vi "configuration UI.vi"() -> ()   [LabVIEW 2013, in "TEC editor node.lvclass"]
uses:
  TEC editor node.lvclass
  <vilib>/NI/Configuration Framework/Node/NodeRef.ctl
  <vilib>/NI/Configuration Framework/Node/NISE_CEF_Node.lvclass
  <vilib>/NI/AMC/Message Queue.ctl
  <vilib>/NI/AMC/Message.ctl
  <vilib>/NI/Tools/Keyed Array/KeyedArray.ctl
  <vilib>/NI/Configuration Framework/Node/UserEventRef.ctl
  <vilib>/NI/Configuration Framework/Controls/EventCluster.ctl
  <vilib>/NI/DCAF UI Toolkit/Controls/Move One Right.ctl
  <vilib>/NI/DCAF UI Toolkit/Controls/Move One Left.ctl
  configuration/TEC configuration.lvclass
  <vilib>/Utility/miscctls.llb/LVRowAndColumnTypeDef.ctl
  <vilib>/Utility/miscctls.llb/LVPositionTypeDef.ctl
  configuration/TEC configuration.lvclass/TEC configuration.ctl
  TEC editor node.lvclass/TEC editor node.ctl
  <vilib>/NI/Tag Bus/tag/Data Type.ctl
  <vilib>/NI/Tag Bus Module Framework/channel/channel classification.ctl
  <vilib>/NI/Tag Bus Module Framework/channel/TBM channel.lvclass/TBM channel.ctl
  <vilib>/NI/Configuration Framework/serializable configuration/NISE_CEF_serializable configuration.lvclass/NISE_CEF_serializable configuration.ctl
  <vilib>/NI/Tag Bus/tag/tag descriptor.lvclass/tag descriptor.ctl
  configuration/Write receive on port.vi
  configuration/Write send to port.vi
  configuration/Write send from port.vi
  configuration/Write send to address.vi
  configuration/Write estimated array size.vi
  configuration/Read receive on port.vi
  configuration/Read send from port.vi
  configuration/Read send to address.vi
  configuration/Read send to port.vi
  configuration/Read estimated array size.vi
  <vilib>/NI/DCAF/Tag Editor Core/Configuration Editor/Classes/Module editor node/Read display name.vi
  <vilib>/Utility/LVClass/Get LV Class Name.vi
  <vilib>/NI/Configuration Framework/error generator/NISE_error generator.vi
  <vilib>/NI/Configuration Framework/serializable configuration/NISE_CEF_serializable configuration.lvclass
  <vilib>/NI/DCAF/Tag Editor Core/Configuration Editor/Classes/Module editor node/module editor node.lvclass
  <vilib>/NI/Configuration Framework/NISE_CEF_TreeControl.lvlib
  <vilib>/NI/Tag Bus/tag/tag descriptor.lvclass
  <vilib>/NI/Module Execution Interface/Engine Configuration/engine configuration.lvclass
  <vilib>/NI/Tag Bus Module Framework/channel/TBM channel.lvclass
  <vilib>/NI/DCAF/Tag Editor Core/Configuration Editor/Classes/Engine Parent/Engine Parent Editor Node.lvclass
  <vilib>/NI/DCAF UI Toolkit/Controls/DCAF UI Elements.lvlib
  <vilib>/NI/Tools/Keyed Array/Tools_KeyedArray.lvlib
  <vilib>/NI/AMC/AMC.lvlib
panel:
  in  "Tab Control":T1(tab)
  out "Guid":string
  in  "unpair":bool
  out "Paired with":string
  in  "pair":bool
  in  "Pairing Options":i32(listbox)
  in  "Filtering":string
  in  "remove to":T2
  in  "add to":T3
  in  "toExtList":i32(listbox)
  in  "fromExternallist":i32(listbox)
  in  "avail tags":i32(listbox)=-1
  in  "Estimated Received Array Size (bytes)":u16
  in  "receive on port":u16
  in  "send from port":u16
  in  "send to address":string
  in  "send to port":u16
  in  "user event":T4
  in  "main queue":T5
  in  "node ref":T6
  # "UDP Port Settings"
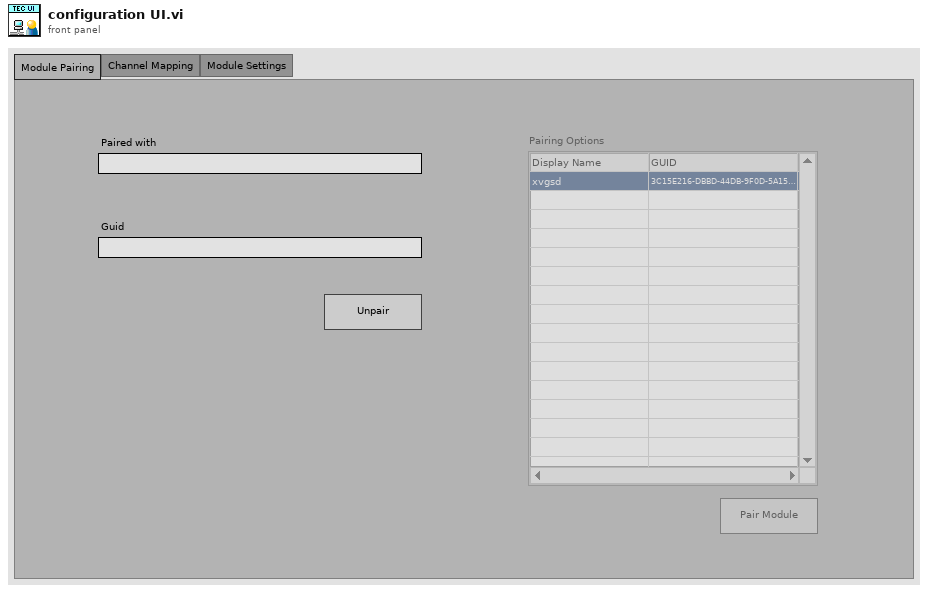
[diagram p1: front panel]
types:
  T1 = enum32{"Module Pairing", "Channel Mapping", "Module Settings"}
  T2 = typedef "DCAF UI Elements.lvlib/Move One Left.ctl" = bool
  T3 = typedef "DCAF UI Elements.lvlib/Move One Right.ctl" = bool
  T4 = typedef "NISE_CEF_Node.lvclass/UserEventRef.ctl" = refnum<user-event>
  T5 = typedef "AMC.lvlib/Message Queue.ctl" = refnum<queue>
  T6 = typedef "NISE_CEF_Node.lvclass/NodeRef.ctl" = refnum<data-value>
  T7 = typedef "LVPositionTypeDef.ctl" = cluster{"Left":i32, "Top":i32}
  T8 = typedef "LVRowAndColumnTypeDef.ctl" = cluster{"Row":i32, "Column":i32}
  T9 = typedef "NISE_CEF_TreeControl.lvlib/EventCluster.ctl" = cluster{"command":string, "data":string}
  T10 = typedef "TBM channel.lvclass/channel classification.ctl" = enum16{"input data", "output data", "processing parameter", "processing result"}
  T11 = typedef "tag bus.lvlib/tag descriptor.lvclass/Data Type.ctl" = enum16{"Double", "Single", "I64", "I32", "I16", "I8", "U64", "U32", "U16", "U8", "Boolean", "String", "Array of Double", "Array of Single", "Array of I64", "Array of I32", "Array of I16", "Array of I8", "Array of U64", "Array of U32", "Array of U16", "Array of U8", "Array of Boolean", "Array of String"}
  T12 = typedef "TEC editor node.lvclass/pair information.ctl" = cluster{"paired guid":string}
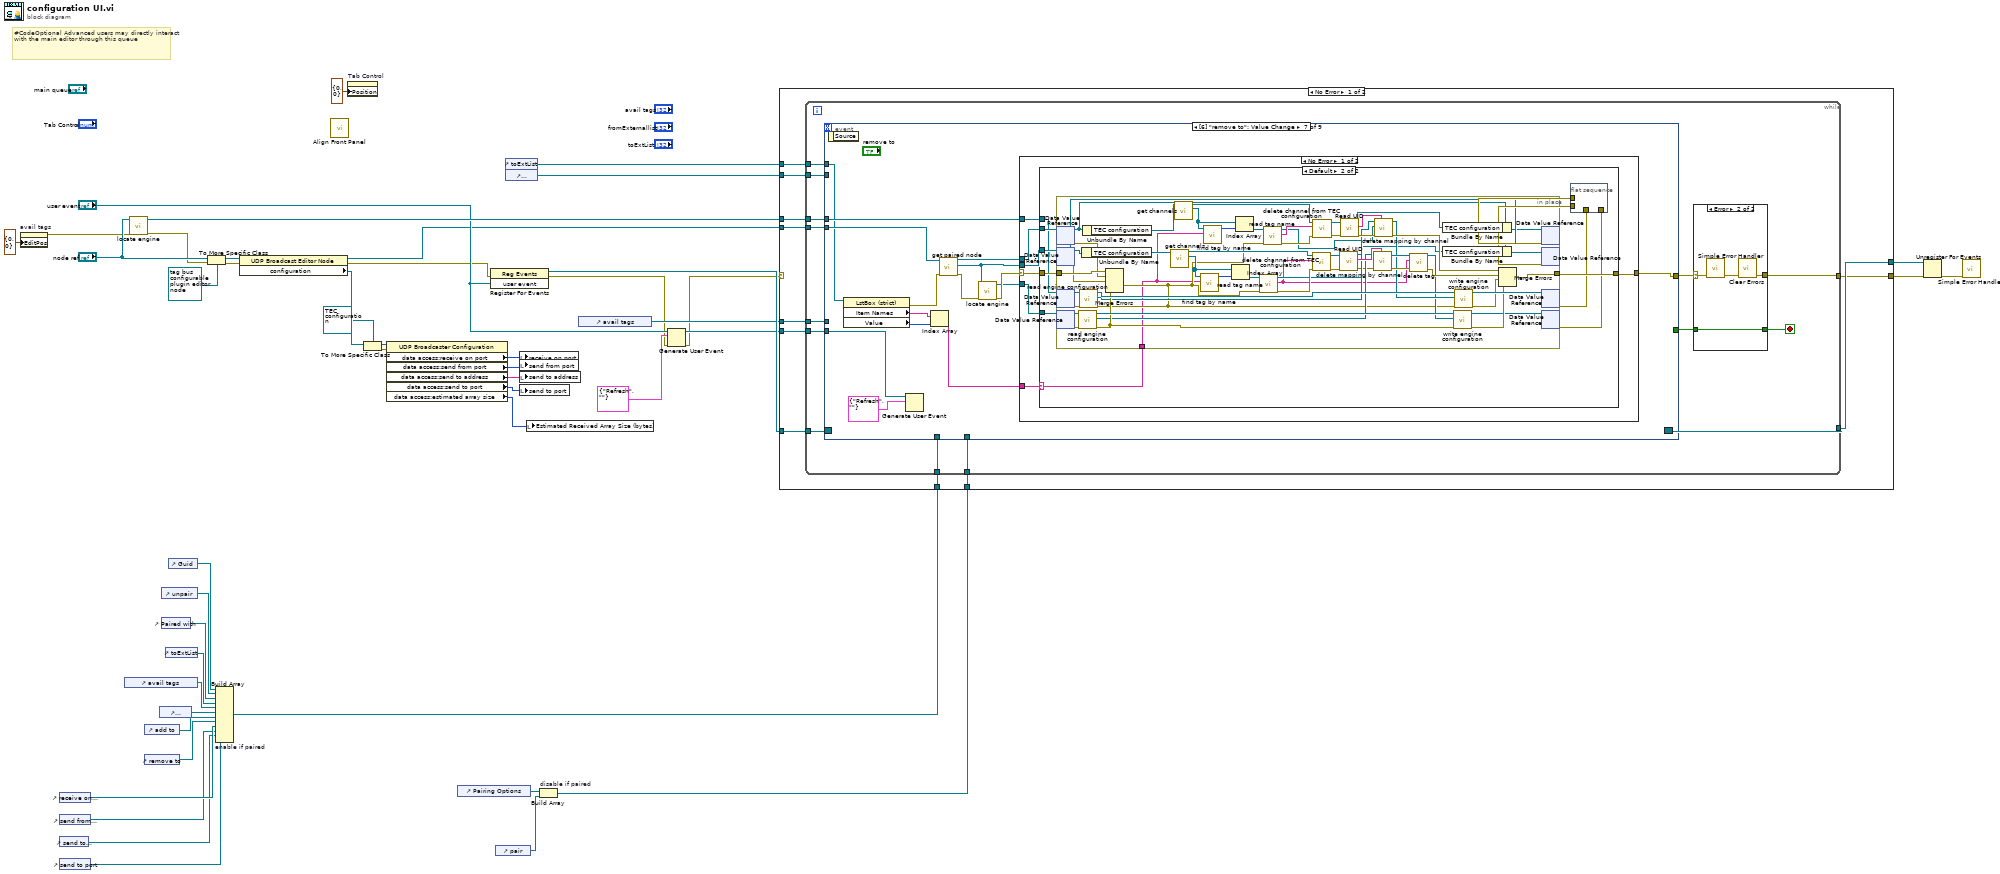
[diagram p0: block diagram]
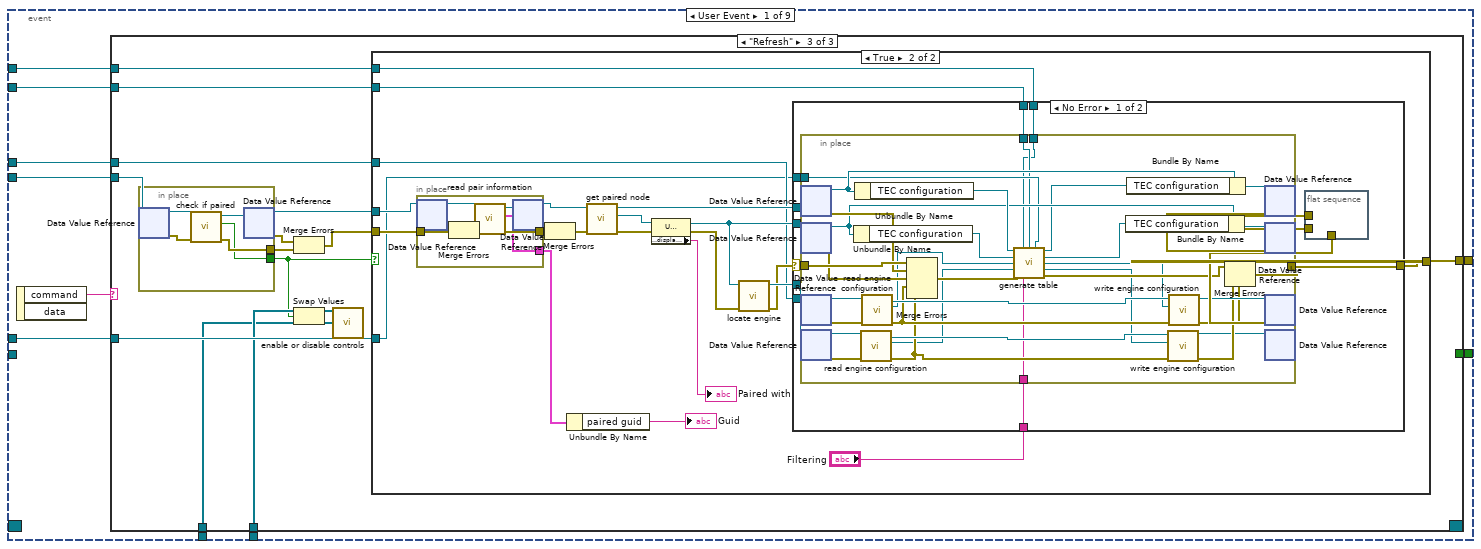
[diagram p3: hidden frame]
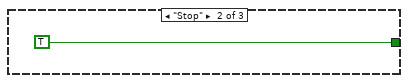
[diagram p5: hidden frame]
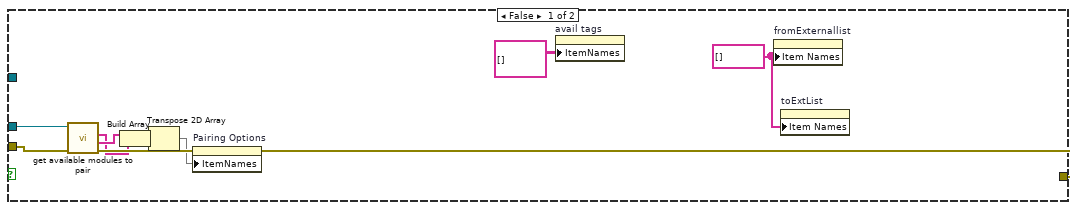
[diagram p6: hidden frame]
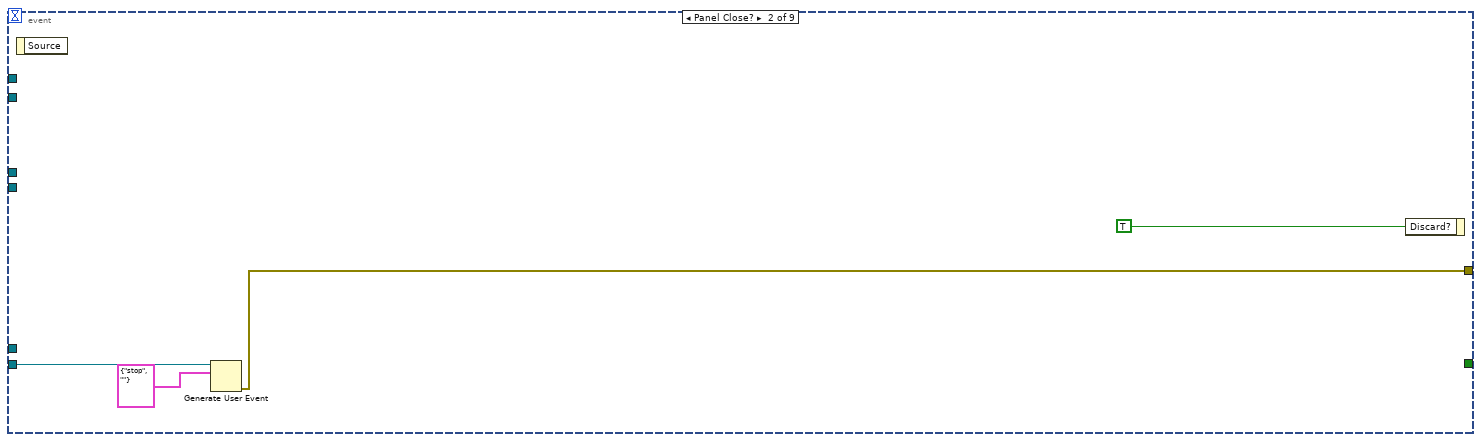
[diagram p8: hidden frame]
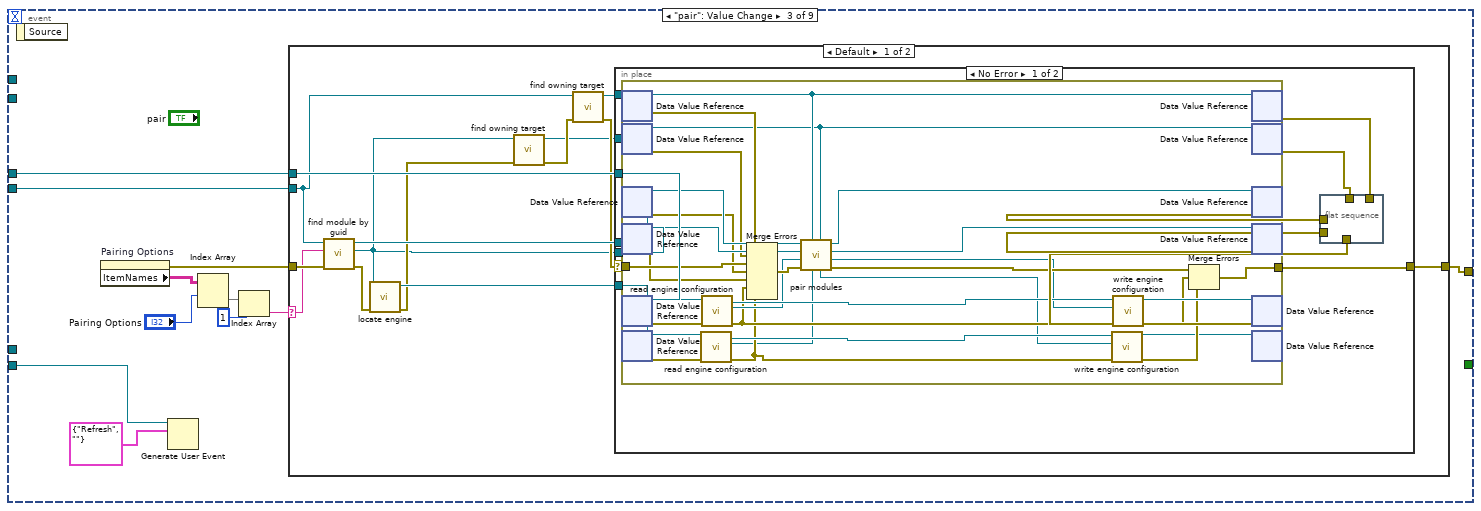
[diagram p9: hidden frame]
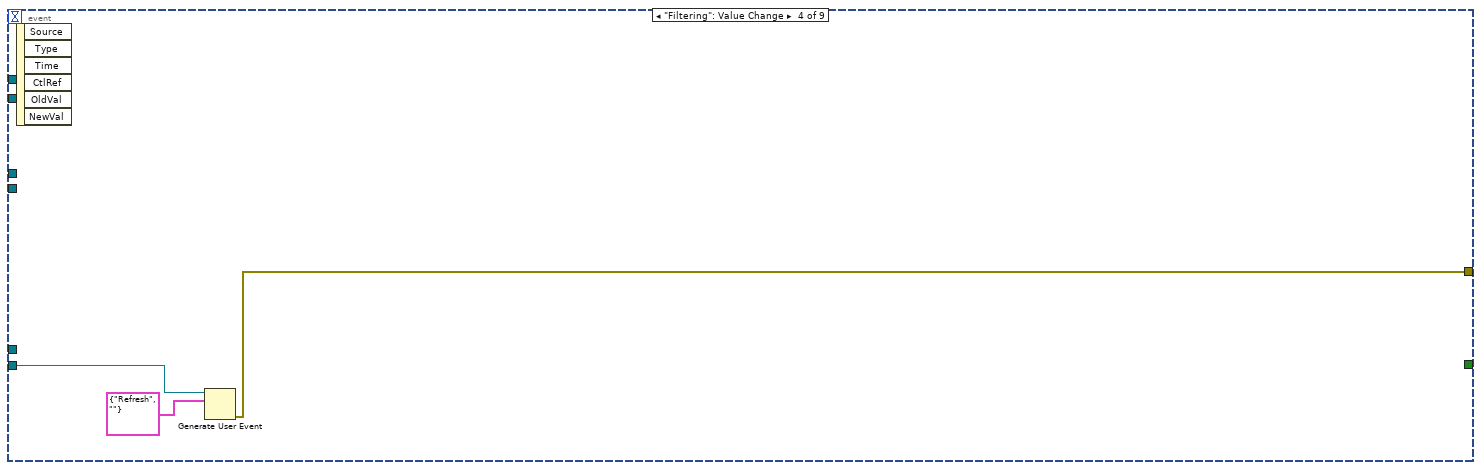
[diagram p12: hidden frame]
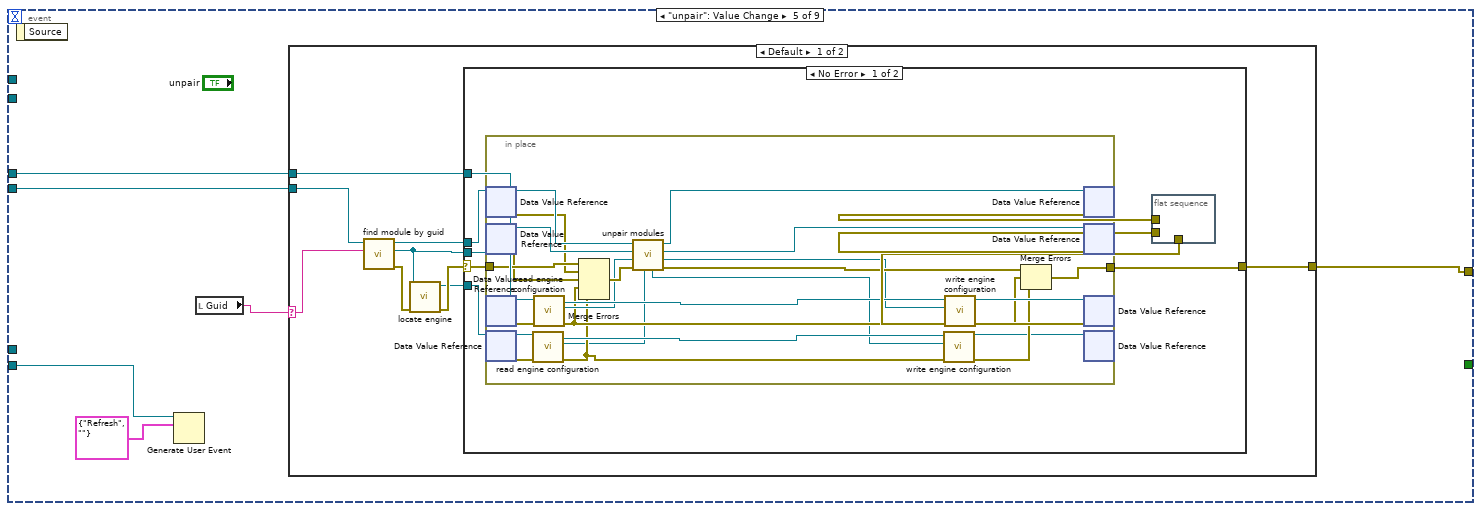
[diagram p13: hidden frame]
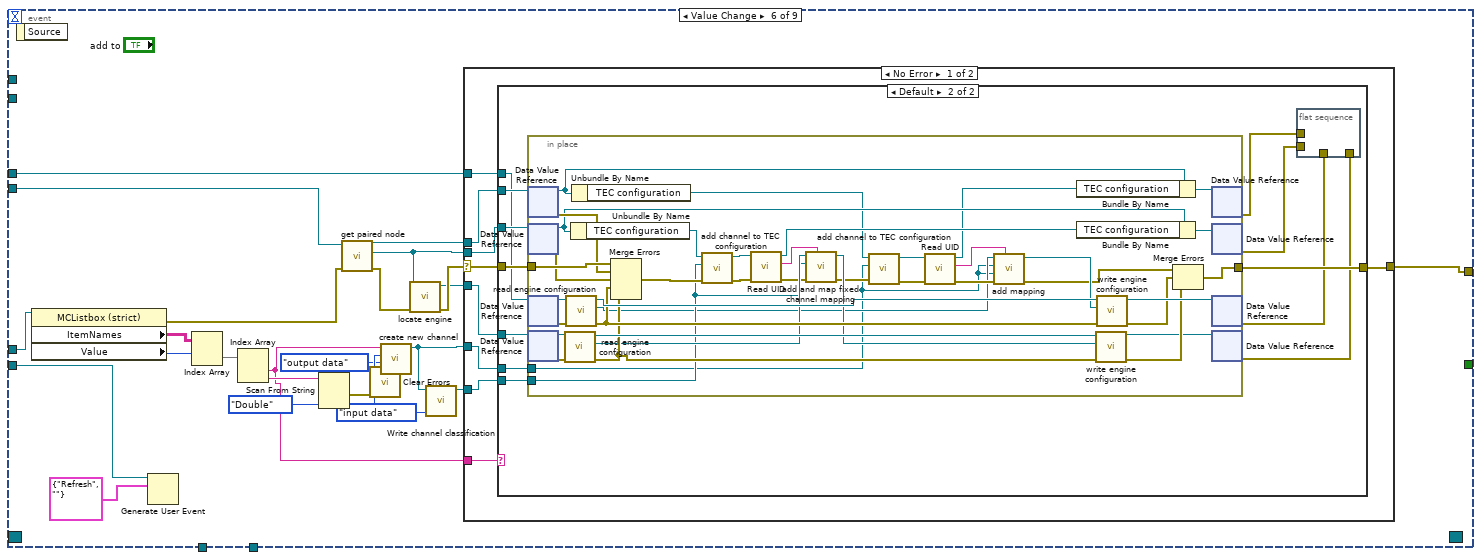
[diagram p16: hidden frame]
diagram:
  # "#CodeOptional Advanced users may directly interact with the main editor through this queue"
  n1 = property on="avail tags" class="MCListbox (strict)"("EditPos"=T8 {"Row"=0, "Column"=0} ("Edit Position")) -> (error out=w4:errorcluster)  [unwired: 2 in, 1 out]
  n2 = control-ref of="receive on port"() -> (w8:refnum<vi>)
  n3 = control-ref of="send from port"() -> (w7:refnum<vi>)
  n4 = control-ref of="send to address"() -> (w6:refnum<vi>)
  n5 = control-ref of="send to port"() -> (w5:refnum<vi>)
  n6 = control-ref of="avail tags"() -> (w29:refnum<vi>)
  n7 = call <vilib>:"locate engine.vi"("error in"=w4, "component"="node ref") -> ("error out"=w34:errorcluster, "engine"=w42:refnum<data-value>)  [unwired: 8 in]
  n8 = control-ref of="add to"() -> (w26:refnum<vi>)
  n9 = control-ref of="remove to"() -> (w27:refnum<vi>)
  n10 = control-ref of="fromExternallist"() -> (w28:refnum<vi>)
  n11 = control-ref of="unpair"() -> (w32:refnum<vi>)
  n12 = control-ref of="Paired with"() -> (w33:refnum<vi>)
  n13 = control-ref of="toExtList"() -> (w30:refnum<vi>)
  n14 = control-ref of="Guid"() -> (w31:refnum<vi>)
  n15 = To More Specific Class(target class=refnum<data-value> refnum ("data value reference"), reference="node ref", error in=w34) -> (specific class reference=w18:refnum<data-value>, error out=w44:errorcluster)
  n16 = Build Array "enable if paired"(w31, w32, w33, w30, w29, w28, w26, w27, w8, w7, w6, w5) -> (w24:refnum<vi>[])
  n17 = property class="UDP Broadcast Editor Node"(reference=w18, error in=w44) -> (reference out=w17:refnum<data-value>, error out=w19:errorcluster, "configuration"=w12:refnum<class "NISE_CEF_serializable configuration.lvclass">)
  n18 = call <vilib>:"Align Front Panel.vi"() -> ()  [unwired: 10 in, 2 out]
  n19 = property on="Tab Control" class="TabCtl (strict)"("Position"=T7 {"Left"=0, "Top"=0}) -> ()  [unwired: 2 in, 2 out]
  n20 = To More Specific Class(target class=refnum<class "TEC configuration.lvclass"> refnum ("UDP Broadcaster Configuration"), reference=w12) -> (specific class reference=w11:refnum<class "TEC configuration.lvclass">, error out=w10:errorcluster)  [unwired: 1 in]
  n21 = property class="UDP Broadcaster Configuration"(reference=w11, error in=w10) -> ("data access:receive on port"=w13:u16, "data access:send from port"=w14:u16, "data access:send to address"=w15:string, "data access:send to port"=w16:u16, "data access:estimated array size"=w2:u16)  [unwired: 2 out]
  n22 = control-ref of="Pairing Options"() -> (w25:refnum<vi>)
  n23 = register-events(error in=w19, "user event") -> (reference out=w48:refnum<event-registration>, error out=w21:errorcluster)  [unwired: 1 in]
  n24 = control-ref of="pair"() -> (w22:refnum<vi>)
  n25 = control-ref of="toExtList"() -> (w40:refnum<vi>)
  n26 = control-ref of="fromExternallist"() -> (w20:refnum<vi>)
  n27 = local write "receive on port"(w13) -> ()
  n28 = local write "send from port"(w14) -> ()
  n29 = local write "send to address"(w15) -> ()
  n30 = local write "send to port"(w16) -> ()
  n31 = local write "Estimated Received Array Size (bytes)"(w2) -> ()
  n32 = Build Array "disable if paired"(w25, w22) -> (w23:refnum<vi>[])
  n33 = control-ref of="avail tags"() -> (w41:refnum<vi>)
  n34 = Generate User Event(user event="user event", event data cluster=T9 {"command"="Refresh", "data"=""} ("event data"), error in=w21) -> (user event out=w38:T4, error out=w36:errorcluster)  [unwired: 1 in]
  n35 = case shown="No Error" w36 {
    selector: w36 -> [_ w544]
    tunnel: w48 -> [w59 w543]
    tunnel: [w58 w543] -> w47
    tunnel: [w57 w544] -> w46
    tunnel: w17 -> [w56 _]
    tunnel: w42 -> [w55 _]
    tunnel: w41 -> [w54 _]
    tunnel: w40 -> [w53 _]
    tunnel: w38 -> [w52 _]
    tunnel: w24 -> [w51 _]
    tunnel: w23 -> [w50 _]
    tunnel: w20 -> [w49 _]
    frame No Error {
      n36 = while {
        tunnel: w59 -> [w73]
        tunnel: [w72] -> w58
        tunnel: w56 -> [w67]
        tunnel: w55 -> [w66]
        tunnel: w52 -> [w65]
        tunnel: w54 -> [w64]
        tunnel: w53 -> [w63]
        tunnel: [w68] -> w57
        tunnel: w51 -> [w62]
        tunnel: w50 -> [w61]
        tunnel: w49 -> [w60]
        stop <- w70 stop-if-true
        n37 = event shown="[6] \"remove to\": Value Change" {
          selector: w73 -> [_ _ _ _ _ _ _ _ _]
          dyn-events: [_ _ _ _ _ _ _ _ _] -> w72
          timeout: _ -> [_ _ _ _ _ _ _ _ _]
          tunnel: [w89 _ _ _ _ _ _ _ _] -> w69
          tunnel: [w87 w198 w205 w272 w279 w349 w428 w508 w535] -> w71
          tunnel: w67 -> [w86 _ w207 _ w280 w345 w424 w507 w534]
          tunnel: w66 -> [w85 _ w204 _ w278 w348 w427 _ _]
          tunnel: w65 -> [_ w199 w202 w273 w275 w340 w419 _ _]
          tunnel: w64 -> [w84 _ _ _ _ w334 _ _ _]
          tunnel: w63 -> [w83 _ _ _ _ _ w416 _ _]
          tunnel: w62 -> [w82 _ _ _ _ _ _ _ _]
          tunnel: w61 -> [w81 _ _ _ _ _ _ _ _]
          tunnel: w60 -> [w80 _ _ _ _ _ _ _ _]
          event User Event {
            n38 = event-data() -> ("command"=w88:string)  [unwired: 1 in, 1 out]
            n39 = case shown="\"Refresh\"" w88 {
              tunnel: [_ TRUE _] -> w89
              tunnel: [_ _ w102] -> w87
              tunnel: w86 -> [_ _ w101]
              tunnel: w85 -> [_ _ w103]
              tunnel: w84 -> [_ _ w105]
              tunnel: w83 -> [_ _ w104]
              tunnel: w82 -> [_ _ w95]
              tunnel: w81 -> [_ _ w96]
              tunnel: w80 -> [_ _ w91]
              frame Default {
              }
              frame "Stop" {
              }
              frame "Refresh" {
                n40 = in-place {
                  in-place-border: [w194] -> w98
                  in-place-border: [w193] -> w92
                  n41 = in-place-dvr #1(w101) -> (w197:refnum<class "TEC editor node.lvclass">, w195:errorcluster)
                  n42 = call "check if paired.vi"("error in"=w195, "UDP Broadcast Editor Node in"=w197) -> ("error out"=w194:errorcluster, "paired"=w193:bool, "UDP Broadcast Editor Node out"=w196:refnum<class "TEC editor node.lvclass">)  [unwired: 7 in]
                  n43 = in-place-dvr #1(w196) -> (w100:refnum<data-value>, w99:errorcluster)
                }
                n44 = Merge Errors(w99, w98) -> (w93:errorcluster)
                n45 = Swap Values(12:w96, 13:w92, 14:w95) -> (1:w97:refnum<vi>[], 3:w94:refnum<vi>[])
                n46 = call "enable or disable controls.vi"("disable set"=w94, "enable set"=w97) -> ()  [unwired: 10 in]
                n47 = case shown="True" w92 {
                  tunnel: w105 -> [_ w117]
                  tunnel: w104 -> [_ w118]
                  tunnel: w103 -> [_ w120]
                  tunnel: [w111 w124] -> w102
                  tunnel: w100 -> [w115 w127]
                  tunnel: w93 -> [w114 w128]
                  tunnel: w91 -> [_ w119]
                  frame False {
                    w106 = string[] [] ("Item Names")
                    n48 = call "get available modules to pair.vi"("error in"=w114, "editor in"=w115) -> ("error out"=w113:errorcluster, "Display Name"=w109:string[], "IDs"=w108:string[])  [unwired: 6 in, 1 out]
                    n49 = Build Array(w109, w108) -> (w112:string[][])
                    n50 = Transpose 2D Array(2D array=w112) -> (transposed array=w110:string[][])
                    n51 = property on="Pairing Options" class="MCListbox (strict)"(error in=w113, "ItemNames"=w110) -> (error out=w111:errorcluster)  [unwired: 1 in, 1 out]
                    n52 = property on="avail tags" class="MCListbox (strict)"("ItemNames"=string[][] [] ("Item Names")) -> ()  [unwired: 2 in, 2 out]
                    n53 = property on="fromExternallist" class="LstBox (strict)"("Item Names"=w106) -> ()  [unwired: 2 in, 2 out]
                    n54 = property on="toExtList" class="LstBox (strict)"("Item Names"=w106) -> ()  [unwired: 2 in, 2 out]
                  }
                  frame True {
                    n55 = in-place {
                      in-place-border: w128 -> [w188]
                      in-place-border: [w192] -> w135
                      in-place-border: [w186] -> w130
                      n56 = in-place-dvr #2(w127) -> (w191:refnum<class "TEC editor node.lvclass">, w187:errorcluster)
                      n57 = Merge Errors(w188, w187) -> (w189:errorcluster)
                      n58 = call "read pair information.vi"("error in"=w189, "UDP Broadcast Editor Node in"=w191) -> ("error out"=w192:errorcluster, "pair info"=w186:T12, "UDP Broadcast Editor Node out"=w190:refnum<class "TEC editor node.lvclass">)  [unwired: 7 in]
                      n59 = in-place-dvr #2(w190) -> (w137:refnum<data-value>, w134:errorcluster)
                    }
                    n60 = Merge Errors(w135, w134) -> (w136:errorcluster)
                    n61 = Unbundle By Name(w130) -> ("paired guid"=→"Guid":string)
                    n62 = call "get paired node.vi"("error in"=w136, "editor in"=w137) -> ("error out"=w132:errorcluster, "paired node"=w133:refnum<data-value>, "editor out"=w122:refnum<data-value>)  [unwired: 7 in]
                    n63 = property class="UDP Broadcast Editor Node"(reference=w133, error in=w132) -> (reference out=w121:refnum<data-value>, error out=w123:errorcluster, "Data Access:display name"=→"Paired with":string)
                    n64 = call <vilib>:"locate engine.vi"("error in"=w123, "component"=w121) -> ("error out"=w125:errorcluster, "engine"=w126:refnum<data-value>)  [unwired: 8 in]
                    n65 = case shown="No Error" w125 {
                      selector: w125 -> [w150 w185]
                      tunnel: [w149 w185] -> w124
                      tunnel: w126 -> [w145 _]
                      tunnel: w122 -> [w144 _]
                      tunnel: w121 -> [w143 _]
                      tunnel: w120 -> [w142 _]
                      tunnel: w119 -> [w141 _]
                      tunnel: w118 -> [w140 _]
                      tunnel: w117 -> [w139 _]
                      tunnel: "Filtering" -> [w138 _]
                      frame No Error {
                        n66 = in-place {
                          in-place-border: w150 -> [w184]
                          in-place-border: [w177] -> w149
                          in-place-border: w141 -> [w153]
                          in-place-border: w140 -> [w152]
                          in-place-border: w139 -> [w154]
                          in-place-border: w138 -> [w151]
                          n67 = in-place-dvr #3(w144) -> (w160:refnum<class "TEC editor node.lvclass">, w183:errorcluster)
                          n68 = in-place-dvr #4(w143) -> (w157:refnum<class "TEC editor node.lvclass">, w182:errorcluster)
                          n69 = in-place-dvr #5(w142) -> (w181:refnum<class "Engine Parent Editor Node.lvclass">, w180:errorcluster)
                          n70 = in-place-dvr #6(w145) -> (w173:refnum<class "Engine Parent Editor Node.lvclass">, w172:errorcluster)
                          n71 = Unbundle By Name(w157) -> ("TEC configuration"=w161:refnum<class "TEC configuration.lvclass">)
                          n72 = Unbundle By Name(w160) -> ("TEC configuration"=w162:refnum<class "TEC configuration.lvclass">)
                          n73 = call <vilib>:"read engine configuration.vi"("error in"=w172, "Engine Parent Editor Node in"=w173) -> ("error out"=w171:errorcluster, "engine configuration"=w164:refnum<class "engine configuration.lvclass">, "Engine Parent Editor Node out"=w174:refnum<class "Engine Parent Editor Node.lvclass">)  [unwired: 7 in]
                          n74 = call <vilib>:"read engine configuration.vi"("error in"=w180, "Engine Parent Editor Node in"=w181) -> ("error out"=w175:errorcluster, "engine configuration"=w163:refnum<class "engine configuration.lvclass">, "Engine Parent Editor Node out"=w179:refnum<class "Engine Parent Editor Node.lvclass">)  [unwired: 7 in]
                          n75 = Merge Errors(w184, w183, w182, w175, w171) -> (w168:errorcluster)
                          n76 = call "generate table.vi"("TEC in"=w162, "from TEC"=w152, "to TEC"=w153, "avail tags"=w154, "Pair in"=w161, "engine configuration in"=w163, "paired engine in"=w164, "error in"=w168, "Filtering"=w151) -> ("TEC out"=w155:refnum<class "TEC configuration.lvclass">, "pair out"=w156:refnum<class "TEC configuration.lvclass">, "engine configuration out"=w165:refnum<class "engine configuration.lvclass">, "paired engine out"=w166:refnum<class "engine configuration.lvclass">, "error out"=w167:errorcluster)  [unwired: 2 in]
                          n77 = Bundle By Name(cluster=w157, "TEC configuration"=w156) -> (w158:refnum<class "TEC editor node.lvclass">)
                          n78 = Bundle By Name(cluster=w160, "TEC configuration"=w155) -> (w159:refnum<class "TEC editor node.lvclass">)
                          n79 = call <vilib>:"write engine configuration.vi"("error in"=w171, "engine configuration"=w166, "Engine Parent Editor Node in"=w174) -> ("error out"=w170:errorcluster, "Engine Parent Editor Node out"=w169:refnum<class "Engine Parent Editor Node.lvclass">)  [unwired: 7 in]
                          n80 = call <vilib>:"write engine configuration.vi"("error in"=w175, "engine configuration"=w165, "Engine Parent Editor Node in"=w179) -> ("error out"=w176:errorcluster, "Engine Parent Editor Node out"=w178:refnum<class "Engine Parent Editor Node.lvclass">)  [unwired: 7 in]
                          n81 = Merge Errors(w167, w176, w170) -> (w177:errorcluster)
                          n82 = in-place-dvr #3(w159) -> (w148:errorcluster)  [unwired: 1 out]
                          n83 = in-place-dvr #4(w158) -> (w147:errorcluster)  [unwired: 1 out]
                          n84 = in-place-dvr #5(w178) -> (w146:errorcluster)  [unwired: 1 out]
                          n85 = in-place-dvr #6(w169) -> ()  [unwired: 2 out]
                        }
                        n86 = flat-sequence {
                          tunnel: w148 -> [_]
                          tunnel: w147 -> [_]
                          tunnel: w146 -> [_]
                          frame #0 {
                          }
                        }
                      }
                      frame Error {
                      }
                    }
                  }
                }
              }
            }
          }
          event Panel Close? {
            n87 = event-data() -> ()  [unwired: 1 in, 1 out]
            n88 = Generate User Event(user event=w199, event data cluster=T9 {"command"="stop", "data"=""} ("event data")) -> (error out=w198:errorcluster)  [unwired: 2 in, 1 out]
            n89 = event-data("Discard?"=TRUE) -> ()  [unwired: 1 in, 1 out]
          }
          event "pair": Value Change {
            n90 = event-data() -> ()  [unwired: 1 in, 1 out]
            n91 = property on="Pairing Options" class="MCListbox (strict)"() -> (error out=w206:errorcluster, "ItemNames"=w212:string[][])  [unwired: 2 in, 1 out]
            n92 = Generate User Event(user event=w202, event data cluster=T9 {"command"="Refresh", "data"=""} ("event data")) -> ()  [unwired: 2 in, 2 out]
            n93 = Index Array(array=w212, index (row)="Pairing Options") -> (element=w210:string[])  [unwired: 1 in]
            n94 = Index Array(array=w210, index=1) -> (element=w208:string)
            n95 = case shown="Default" w208 {
              selector: w208 -> [w225 _]
              tunnel: w207 -> [w215 _]
              tunnel: w206 -> [w226 w271]
              tunnel: [w224 w271] -> w205
              tunnel: w204 -> [w222 _]
              frame Default {
                n96 = call "find module by guid.vi"("error in (no error)"=w226, "GUID"=w225, "ME in"=w215) -> ("error out"=w221:errorcluster, "UDP refs"=w214:refnum<data-value>, "ME out"=w223:refnum<data-value>)  [unwired: 6 in]
                n97 = call <vilib>:"locate engine.vi"("error in"=w221, "component"=w214) -> ("error out"=w216:errorcluster, "engine"=w220:refnum<data-value>)  [unwired: 8 in]
                n98 = call "find owning target.vi"("error in"=w216, "node"=w214) -> ("error out"=w218:errorcluster, "target"=w213:refnum<data-value>)  [unwired: 8 in]
                n99 = call "find owning target.vi"("error in"=w218, "node"=w215) -> ("error out"=w217:errorcluster, "target"=w219:refnum<data-value>)  [unwired: 8 in]
                n100 = case shown="No Error" w217 {
                  selector: w217 -> [w239 w270]
                  tunnel: [w238 w270] -> w224
                  tunnel: w223 -> [w237 _]
                  tunnel: w214 -> [w236 _]
                  tunnel: w222 -> [w235 _]
                  tunnel: w220 -> [w231 _]
                  tunnel: w219 -> [w230 _]
                  tunnel: w213 -> [w229 _]
                  frame No Error {
                    n101 = in-place {
                      in-place-border: w239 -> [w269]
                      in-place-border: [w254] -> w238
                      n102 = in-place-dvr #7(w230) -> (w241:refnum<class "Targets.lvclass">, w243:errorcluster)
                      n103 = in-place-dvr #8(w229) -> (w240:refnum<class "Targets.lvclass">, w242:errorcluster)
                      n104 = in-place-dvr #9(w237) -> (w266:refnum<class "TEC editor node.lvclass">, w264:errorcluster)
                      n105 = in-place-dvr #10(w236) -> (w267:refnum<class "TEC editor node.lvclass">, w263:errorcluster)
                      n106 = in-place-dvr #11(w235) -> (w260:refnum<class "Engine Parent Editor Node.lvclass">, w259:errorcluster)
                      n107 = in-place-dvr #12(w231) -> (w250:refnum<class "Engine Parent Editor Node.lvclass">, w249:errorcluster)
                      n108 = call <vilib>:"read engine configuration.vi"("error in"=w249, "Engine Parent Editor Node in"=w250) -> ("error out"=w248:errorcluster, "engine configuration"=w244:refnum<class "engine configuration.lvclass">, "Engine Parent Editor Node out"=w251:refnum<class "Engine Parent Editor Node.lvclass">)  [unwired: 7 in]
                      n109 = call <vilib>:"read engine configuration.vi"("error in"=w259, "Engine Parent Editor Node in"=w260) -> ("error out"=w252:errorcluster, "engine configuration"=w256:refnum<class "engine configuration.lvclass">, "Engine Parent Editor Node out"=w258:refnum<class "Engine Parent Editor Node.lvclass">)  [unwired: 7 in]
                      n110 = Merge Errors(w243, w242, w269, w264, w263, w252, w248) -> (w265:errorcluster)
                      n111 = call "pair modules.vi"("paired target in"=w240, "paired engine in"=w244, "target in"=w241, "error in"=w265, "engine configuration in"=w256, "module to pair with"=w267, "UDP Broadcast Editor Node in"=w266) -> ("error out"=w268:errorcluster, "engine configuration out"=w255:refnum<class "engine configuration.lvclass">, "module to pair with out"=w261:refnum<class "TEC editor node.lvclass">, "UDP Broadcast Editor Node out"=w262:refnum<class "TEC editor node.lvclass">, "paired engine out"=w245:refnum<class "engine configuration.lvclass">)
                      n112 = call <vilib>:"write engine configuration.vi"("error in"=w248, "engine configuration"=w245, "Engine Parent Editor Node in"=w251) -> ("error out"=w247:errorcluster, "Engine Parent Editor Node out"=w246:refnum<class "Engine Parent Editor Node.lvclass">)  [unwired: 7 in]
                      n113 = call <vilib>:"write engine configuration.vi"("error in"=w252, "engine configuration"=w255, "Engine Parent Editor Node in"=w258) -> ("error out"=w253:errorcluster, "Engine Parent Editor Node out"=w257:refnum<class "Engine Parent Editor Node.lvclass">)  [unwired: 7 in]
                      n114 = Merge Errors(w268, w253, w247) -> (w254:errorcluster)
                      n115 = in-place-dvr #7(w241) -> (w227:errorcluster)  [unwired: 1 out]
                      n116 = in-place-dvr #8(w240) -> (w228:errorcluster)  [unwired: 1 out]
                      n117 = in-place-dvr #9(w262) -> (w234:errorcluster)  [unwired: 1 out]
                      n118 = in-place-dvr #10(w261) -> (w233:errorcluster)  [unwired: 1 out]
                      n119 = in-place-dvr #11(w257) -> (w232:errorcluster)  [unwired: 1 out]
                      n120 = in-place-dvr #12(w246) -> ()  [unwired: 2 out]
                    }
                    n121 = flat-sequence {
                      tunnel: w234 -> [_]
                      tunnel: w233 -> [_]
                      tunnel: w232 -> [_]
                      tunnel: w228 -> [_]
                      tunnel: w227 -> [_]
                      frame #0 {
                      }
                    }
                  }
                  frame Error {
                  }
                }
              }
              frame "" {
                # "do nothing if nothing was selected"
              }
            }
          }
          event "Filtering": Value Change {
            n122 = event-data() -> ()  [unwired: 1 in, 6 out]
            n123 = Generate User Event(user event=w273, event data cluster=T9 {"command"="Refresh", "data"=""} ("event data")) -> (error out=w272:errorcluster)  [unwired: 2 in, 1 out]
          }
          event "unpair": Value Change {
            n124 = event-data() -> ()  [unwired: 1 in, 1 out]
            n125 = Generate User Event(user event=w275, event data cluster=T9 {"command"="Refresh", "data"=""} ("event data")) -> ()  [unwired: 2 in, 2 out]
            n126 = local read "Guid"() -> (w277:string)
            n127 = case shown="Default" w277 {
              selector: w277 -> [w288 _]
              tunnel: w280 -> [w289 _]
              tunnel: [w287 _] -> w279
              tunnel: w278 -> [w285 _]
              frame Default {
                n128 = call "find module by guid.vi"("GUID"=w288, "ME in"=w289) -> ("error out"=w284:errorcluster, "UDP refs"=w282:refnum<data-value>, "ME out"=w286:refnum<data-value>)  [unwired: 7 in]
                n129 = call <vilib>:"locate engine.vi"("error in"=w284, "component"=w282) -> ("error out"=w283:errorcluster, "engine"=w281:refnum<data-value>)  [unwired: 8 in]
                n130 = case shown="No Error" w283 {
                  selector: w283 -> [w298 w325]
                  tunnel: [w297 w325] -> w287
                  tunnel: w286 -> [w296 _]
                  tunnel: w282 -> [w295 _]
                  tunnel: w285 -> [w294 _]
                  tunnel: w281 -> [w290 _]
                  frame No Error {
                    n131 = in-place {
                      in-place-border: w298 -> [w324]
                      in-place-border: [w309] -> w297
                      n132 = in-place-dvr #13(w296) -> (w321:refnum<class "TEC editor node.lvclass">, w319:errorcluster)
                      n133 = in-place-dvr #14(w295) -> (w322:refnum<class "TEC editor node.lvclass">, w318:errorcluster)
                      n134 = in-place-dvr #15(w294) -> (w315:refnum<class "Engine Parent Editor Node.lvclass">, w314:errorcluster)
                      n135 = in-place-dvr #16(w290) -> (w305:refnum<class "Engine Parent Editor Node.lvclass">, w304:errorcluster)
                      n136 = call <vilib>:"read engine configuration.vi"("error in"=w304, "Engine Parent Editor Node in"=w305) -> ("error out"=w303:errorcluster, "engine configuration"=w299:refnum<class "engine configuration.lvclass">, "Engine Parent Editor Node out"=w306:refnum<class "Engine Parent Editor Node.lvclass">)  [unwired: 7 in]
                      n137 = call <vilib>:"read engine configuration.vi"("error in"=w314, "Engine Parent Editor Node in"=w315) -> ("error out"=w307:errorcluster, "engine configuration"=w311:refnum<class "engine configuration.lvclass">, "Engine Parent Editor Node out"=w313:refnum<class "Engine Parent Editor Node.lvclass">)  [unwired: 7 in]
                      n138 = Merge Errors(w324, w319, w318, w307, w303) -> (w320:errorcluster)
                      n139 = call "unpair modules.vi"("paired engine in"=w299, "error in"=w320, "engine configuration in"=w311, "module to unpair"=w322, "UDP Broadcast Editor Node in"=w321) -> ("error out"=w323:errorcluster, "engine configuration out"=w310:refnum<class "engine configuration.lvclass">, "unpaired module"=w316:refnum<class "TEC editor node.lvclass">, "UDP Broadcast Editor Node out"=w317:refnum<class "TEC editor node.lvclass">, "paired engine out"=w300:refnum<class "engine configuration.lvclass">)  [unwired: 2 in]
                      n140 = call <vilib>:"write engine configuration.vi"("error in"=w303, "engine configuration"=w300, "Engine Parent Editor Node in"=w306) -> ("error out"=w302:errorcluster, "Engine Parent Editor Node out"=w301:refnum<class "Engine Parent Editor Node.lvclass">)  [unwired: 7 in]
                      n141 = call <vilib>:"write engine configuration.vi"("error in"=w307, "engine configuration"=w310, "Engine Parent Editor Node in"=w313) -> ("error out"=w308:errorcluster, "Engine Parent Editor Node out"=w312:refnum<class "Engine Parent Editor Node.lvclass">)  [unwired: 7 in]
                      n142 = Merge Errors(w323, w308, w302) -> (w309:errorcluster)
                      n143 = in-place-dvr #13(w317) -> (w293:errorcluster)  [unwired: 1 out]
                      n144 = in-place-dvr #14(w316) -> (w292:errorcluster)  [unwired: 1 out]
                      n145 = in-place-dvr #15(w312) -> (w291:errorcluster)  [unwired: 1 out]
                      n146 = in-place-dvr #16(w301) -> ()  [unwired: 2 out]
                    }
                    n147 = flat-sequence {
                      tunnel: w293 -> [_]
                      tunnel: w292 -> [_]
                      tunnel: w291 -> [_]
                      frame #0 {
                      }
                    }
                  }
                  frame Error {
                  }
                }
              }
              frame "" {
                # "do nothing if nothing was selected"
              }
            }
          }
          event Value Change {
            n148 = event-data() -> ()  [unwired: 1 in, 1 out]
            n149 = property class="MCListbox (strict)"(reference=w334) -> (error out=w327:errorcluster, "ItemNames"=w339:string[][], "Value"=w338:i32)  [unwired: 1 in, 1 out]
            n150 = Generate User Event(user event=w340, event data cluster=T9 {"command"="Refresh", "data"=""} ("event data")) -> ()  [unwired: 2 in, 2 out]
            n151 = Index Array(array=w339, index (row)=w338) -> (element=w335:string[])  [unwired: 1 in]
            n152 = Index Array(array=w335) -> (element #1=w328:string, element #2=w337:string)  [unwired: 2 in]
            n153 = Scan From String(input string=w337, default 1=Data_Type."Double" ("data type")) -> (error out=w326:errorcluster, output 1=w333:T11)  [unwired: 3 in, 2 out]
            n154 = call "get paired node.vi"("error in"=w327, "editor in"=w345) -> ("error out"=w342:errorcluster, "paired node"=w343:refnum<data-value>, "editor out"=w344:refnum<data-value>)  [unwired: 7 in]
            n155 = call <vilib>:"Clear Errors.vi"("error in (no error)"=w326) -> ()  [unwired: 6 in, 1 out]
            n156 = call <vilib>:"create new channel.vi"("channel classification"=channel_classification."output data", "data type"=w333, "channel name"=w328) -> ("channel"=w331:refnum<class "TBM channel.lvclass">)  [unwired: 8 in]
            n157 = call <vilib>:"locate engine.vi"("error in"=w342, "component"=w343) -> ("error out"=w347:errorcluster, "engine"=w346:refnum<data-value>)  [unwired: 8 in]
            n158 = call <vilib>:"Write channel classification.vi"("channel classification"=channel_classification."input data", "channel in"=w331) -> ("channel out"=w330:refnum<class "TBM channel.lvclass">)  [unwired: 8 in, 1 out]
            n159 = case shown="No Error" w347 {
              selector: w347 -> [w358 w413]
              tunnel: [w357 w413] -> w349
              tunnel: w344 -> [w356 _]
              tunnel: w343 -> [w355 _]
              tunnel: w348 -> [w354 _]
              tunnel: w346 -> [w353 _]
              tunnel: w331 -> [w350 _]
              tunnel: w330 -> [w351 _]
              tunnel: w328 -> [w352 _]
              frame No Error {
                n160 = case shown="Default" w352 {
                  tunnel: w358 -> [w359 w371]
                  tunnel: [w359 w370] -> w357
                  tunnel: w356 -> [_ w369]
                  tunnel: w355 -> [_ w368]
                  tunnel: w354 -> [_ w367]
                  tunnel: w353 -> [_ w364]
                  tunnel: w351 -> [_ w361]
                  tunnel: w350 -> [_ w360]
                  frame "" {
                  }
                  frame Default {
                    n161 = in-place {
                      in-place-border: w371 -> [w412]
                      in-place-border: [w405] -> w370
                      in-place-border: w361 -> [w390]
                      in-place-border: w360 -> [w374]
                      n162 = in-place-dvr #17(w369) -> (w395:refnum<class "TEC editor node.lvclass">, w411:errorcluster)
                      n163 = in-place-dvr #18(w368) -> (w394:refnum<class "TEC editor node.lvclass">, w410:errorcluster)
                      n164 = in-place-dvr #19(w367) -> (w409:refnum<class "Engine Parent Editor Node.lvclass">, w408:errorcluster)
                      n165 = in-place-dvr #20(w364) -> (w401:refnum<class "Engine Parent Editor Node.lvclass">, w400:errorcluster)
                      n166 = call <vilib>:"read engine configuration.vi"("error in"=w400, "Engine Parent Editor Node in"=w401) -> ("error out"=w399:errorcluster, "engine configuration"=w391:refnum<class "engine configuration.lvclass">, "Engine Parent Editor Node out"=w402:refnum<class "Engine Parent Editor Node.lvclass">)  [unwired: 7 in]
                      n167 = call <vilib>:"read engine configuration.vi"("error in"=w408, "Engine Parent Editor Node in"=w409) -> ("error out"=w403:errorcluster, "engine configuration"=w376:refnum<class "engine configuration.lvclass">, "Engine Parent Editor Node out"=w407:refnum<class "Engine Parent Editor Node.lvclass">)  [unwired: 7 in]
                      n168 = Unbundle By Name(w394) -> ("TEC configuration"=w392:refnum<class "TEC configuration.lvclass">)
                      n169 = Unbundle By Name(w395) -> ("TEC configuration"=w382:refnum<class "TEC configuration.lvclass">)
                      n170 = Merge Errors(w412, w411, w410, w403, w399) -> (w396:errorcluster)
                      n171 = call "add channel to TEC configuration.vi"("error in"=w396, "channel"=w390, "TEC configuration in"=w392) -> ("error out"=w389:errorcluster, "TEC configuration out"=w388:refnum<class "TEC configuration.lvclass">)  [unwired: 7 in]
                      n172 = call <vilib>:"Read UID.vi"("error in"=w389, "configuration in"=w388) -> ("error out"=w387:errorcluster, "instance id"=w386:string, "configuration out"=w385:refnum<class "TEC configuration.lvclass">)  [unwired: 7 in]
                      n173 = call <vilib>:"add and map fixed channel mapping.vi"("module instance"=w386, "error in"=w387, "fixed channel"=w390, "engine configuration in"=w391) -> ("error out"=w383:errorcluster, "engine configuration out"=w384:refnum<class "engine configuration.lvclass">)  [unwired: 6 in]
                      n174 = call "add channel to TEC configuration.vi"("error in"=w383, "channel"=w374, "TEC configuration in"=w382) -> ("error out"=w380:errorcluster, "TEC configuration out"=w381:refnum<class "TEC configuration.lvclass">)  [unwired: 7 in]
                      n175 = call <vilib>:"Read UID.vi"("error in"=w380, "configuration in"=w381) -> ("error out"=w379:errorcluster, "instance id"=w375:string, "configuration out"=w378:refnum<class "TEC configuration.lvclass">)  [unwired: 7 in]
                      n176 = call <vilib>:"add mapping.vi"("owner ID"=w375, "error in"=w379, "channel"=w374, "tag descriptor"=w374, "engine configuration"=w376) -> ("error out"=w373:errorcluster, "engine configuration out"=w377:refnum<class "engine configuration.lvclass">)  [unwired: 5 in]
                      n177 = Bundle By Name(cluster=w395, "TEC configuration"=w378) -> (w372:refnum<class "TEC editor node.lvclass">)
                      n178 = Bundle By Name(cluster=w394, "TEC configuration"=w385) -> (w393:refnum<class "TEC editor node.lvclass">)
                      n179 = call <vilib>:"write engine configuration.vi"("error in"=w399, "engine configuration"=w384, "Engine Parent Editor Node in"=w402) -> ("error out"=w398:errorcluster, "Engine Parent Editor Node out"=w397:refnum<class "Engine Parent Editor Node.lvclass">)  [unwired: 7 in]
                      n180 = call <vilib>:"write engine configuration.vi"("error in"=w403, "engine configuration"=w377, "Engine Parent Editor Node in"=w407) -> ("error out"=w404:errorcluster, "Engine Parent Editor Node out"=w406:refnum<class "Engine Parent Editor Node.lvclass">)  [unwired: 7 in]
                      n181 = Merge Errors(w373, w404, w398) -> (w405:errorcluster)
                      n182 = in-place-dvr #17(w372) -> (w366:errorcluster)  [unwired: 1 out]
                      n183 = in-place-dvr #18(w393) -> (w365:errorcluster)  [unwired: 1 out]
                      n184 = in-place-dvr #19(w406) -> (w363:errorcluster)  [unwired: 1 out]
                      n185 = in-place-dvr #20(w397) -> (w362:errorcluster)  [unwired: 1 out]
                    }
                    n186 = flat-sequence {
                      tunnel: w366 -> [_]
                      tunnel: w365 -> [_]
                      tunnel: w363 -> [_]
                      tunnel: w362 -> [_]
                      frame #0 {
                      }
                    }
                  }
                }
              }
              frame Error {
              }
            }
          }
          event Value Change {
            n187 = event-data() -> ()  [unwired: 1 in, 1 out]
            n188 = property class="LstBox (strict)"(reference=w416) -> (error out=w415:errorcluster, "Item Names"=w418:string[], "Value"=w417:i32)  [unwired: 1 in, 1 out]
            n189 = Generate User Event(user event=w419, event data cluster=T9 {"command"="Refresh", "data"=""} ("event data")) -> ()  [unwired: 2 in, 2 out]
            n190 = Index Array(array=w418, index=w417) -> (element=w414:string)
            n191 = call "get paired node.vi"("error in"=w415, "editor in"=w424) -> ("error out"=w421:errorcluster, "paired node"=w422:refnum<data-value>, "editor out"=w423:refnum<data-value>)  [unwired: 7 in]
            n192 = call <vilib>:"locate engine.vi"("error in"=w421, "component"=w422) -> ("error out"=w426:errorcluster, "engine"=w425:refnum<data-value>)  [unwired: 8 in]
            n193 = case shown="No Error" w426 {
              selector: w426 -> [w435 w503]
              tunnel: [w434 w503] -> w428
              tunnel: w423 -> [w433 _]
              tunnel: w422 -> [w432 _]
              tunnel: w427 -> [w431 _]
              tunnel: w425 -> [w430 _]
              tunnel: w414 -> [w429 _]
              frame No Error {
                n194 = case shown="Default" w429 {
                  selector: w429 -> [_ w437]
                  tunnel: w435 -> [w436 w447]
                  tunnel: [w436 w446] -> w434
                  tunnel: w433 -> [_ w445]
                  tunnel: w432 -> [_ w444]
                  tunnel: w431 -> [_ w443]
                  tunnel: w430 -> [_ w440]
                  frame "" {
                  }
                  frame Default {
                    n195 = in-place {
                      in-place-border: w447 -> [w502]
                      in-place-border: [w495] -> w446
                      in-place-border: w437 -> [w449]
                      n196 = in-place-dvr #21(w445) -> (w487:refnum<class "TEC editor node.lvclass">, w501:errorcluster)
                      n197 = in-place-dvr #22(w444) -> (w486:refnum<class "TEC editor node.lvclass">, w500:errorcluster)
                      n198 = in-place-dvr #23(w443) -> (w499:refnum<class "Engine Parent Editor Node.lvclass">, w498:errorcluster)
                      n199 = in-place-dvr #24(w440) -> (w492:refnum<class "Engine Parent Editor Node.lvclass">, w491:errorcluster)
                      n200 = call <vilib>:"read engine configuration.vi"("error in"=w491, "Engine Parent Editor Node in"=w492) -> ("error out"=w490:errorcluster, "engine configuration"=w472:refnum<class "engine configuration.lvclass">, "Engine Parent Editor Node out"=w493:refnum<class "Engine Parent Editor Node.lvclass">)  [unwired: 7 in]
                      n201 = call <vilib>:"read engine configuration.vi"("error in"=w498, "Engine Parent Editor Node in"=w499) -> ("error out"=w455:errorcluster, "engine configuration"=w471:refnum<class "engine configuration.lvclass">, "Engine Parent Editor Node out"=w497:refnum<class "Engine Parent Editor Node.lvclass">)  [unwired: 7 in]
                      n202 = Unbundle By Name(w486) -> ("TEC configuration"=w462:refnum<class "TEC configuration.lvclass">)
                      n203 = Unbundle By Name(w487) -> ("TEC configuration"=w460:refnum<class "TEC configuration.lvclass">)
                      n204 = Merge Errors(w502, w501, w500, w455, w490) -> ()  [unwired: 1 out]
                      n205 = call-dynamic "get channels.vi"("TEC configuration in"=w462) -> ("channels"=w464:refnum<class "TBM channel.lvclass">[], "TEC configuration out"=w461:refnum<class "TEC configuration.lvclass">)  [unwired: 9 in]
                      n206 = call-dynamic "get channels.vi"("TEC configuration in"=w460) -> ("channels"=w467:refnum<class "TBM channel.lvclass">[], "TEC configuration out"=w459:refnum<class "TEC configuration.lvclass">)  [unwired: 9 in]
                      n207 = call <vilib>:"find tag by name.vi"("name"=w449, "tags in"=w464) -> ("index"=w463:i32)  [unwired: 9 in]
                      n208 = call <vilib>:"find tag by name.vi"("name"=w449, "tags in"=w467) -> ("index"=w466:i32)  [unwired: 9 in]
                      n209 = Index Array(array=w464, index=w463) -> (element=w465:refnum<class "TBM channel.lvclass">)
                      n210 = Index Array(array=w467, index=w466) -> (element=w468:refnum<class "TBM channel.lvclass">)
                      n211 = call <vilib>:"read tag name.vi"("error in"=w455, "system tag in"=w465) -> ("error out"=w456:errorcluster, "name"=w450:string, "system tag out"=w452:refnum<class "TBM channel.lvclass">)  [unwired: 7 in]
                      n212 = call <vilib>:"read tag name.vi"("error in"=w455, "system tag in"=w468) -> ("error out"=w457:errorcluster, "name"=w458:string, "system tag out"=w453:refnum<class "TBM channel.lvclass">)  [unwired: 7 in]
                      n213 = call "delete channel from TEC configuration.vi"("error in"=w456, "channel to delete"=w450, "TEC configuration in"=w461) -> ("error out"=w454:errorcluster, "TEC configuration out"=w481:refnum<class "TEC configuration.lvclass">)  [unwired: 7 in]
                      n214 = call "delete channel from TEC configuration.vi"("error in"=w457, "channel to delete"=w458, "TEC configuration in"=w459) -> ("error out"=w483:errorcluster, "TEC configuration out"=w484:refnum<class "TEC configuration.lvclass">)  [unwired: 7 in]
                      n215 = call <vilib>:"Read UID.vi"("error in"=w454, "configuration in"=w481) -> ("error out"=w451:errorcluster, "instance id"=w478:string, "configuration out"=w469:refnum<class "TEC configuration.lvclass">)  [unwired: 7 in]
                      n216 = call <vilib>:"Read UID.vi"("error in"=w483, "configuration in"=w484) -> ("error out"=w482:errorcluster, "instance id"=w477:string, "configuration out"=w470:refnum<class "TEC configuration.lvclass">)  [unwired: 7 in]
                      n217 = call <vilib>:"delete mapping by channel.vi"("owner ID"=w478, "error in"=w451, "channel"=w452, "engine configuration in"=w472) -> ("error out"=w479:errorcluster, "engine configuration out"=w480:refnum<class "engine configuration.lvclass">)  [unwired: 6 in]
                      n218 = call <vilib>:"delete mapping by channel.vi"("owner ID"=w477, "error in"=w482, "channel"=w453, "engine configuration in"=w471) -> ("error out"=w475:errorcluster, "engine configuration out"=w474:refnum<class "engine configuration.lvclass">)  [unwired: 6 in]
                      n219 = call <vilib>:"delete tag.vi"("error in"=w479, "tag name"=w450, "engine configuration in"=w480) -> ("error out"=w476:errorcluster, "engine configuration out"=w473:refnum<class "engine configuration.lvclass">)  [unwired: 7 in]
                      n220 = Bundle By Name(cluster=w487, "TEC configuration"=w470) -> (w448:refnum<class "TEC editor node.lvclass">)
                      n221 = Bundle By Name(cluster=w486, "TEC configuration"=w469) -> (w485:refnum<class "TEC editor node.lvclass">)
                      n222 = call <vilib>:"write engine configuration.vi"("error in"=w490, "engine configuration"=w473, "Engine Parent Editor Node in"=w493) -> ("error out"=w489:errorcluster, "Engine Parent Editor Node out"=w488:refnum<class "Engine Parent Editor Node.lvclass">)  [unwired: 7 in]
                      n223 = call <vilib>:"write engine configuration.vi"("error in"=w455, "engine configuration"=w474, "Engine Parent Editor Node in"=w497) -> ("error out"=w494:errorcluster, "Engine Parent Editor Node out"=w496:refnum<class "Engine Parent Editor Node.lvclass">)  [unwired: 7 in]
                      n224 = Merge Errors(w475, w476, w494, w489) -> (w495:errorcluster)
                      n225 = in-place-dvr #21(w448) -> (w442:errorcluster)  [unwired: 1 out]
                      n226 = in-place-dvr #22(w485) -> (w441:errorcluster)  [unwired: 1 out]
                      n227 = in-place-dvr #23(w496) -> (w439:errorcluster)  [unwired: 1 out]
                      n228 = in-place-dvr #24(w488) -> (w438:errorcluster)  [unwired: 1 out]
                    }
                    n229 = flat-sequence {
                      tunnel: w442 -> [_]
                      tunnel: w441 -> [_]
                      tunnel: w439 -> [_]
                      tunnel: w438 -> [_]
                      frame #0 {
                      }
                    }
                  }
                }
              }
              frame Error {
              }
            }
          }
          event "receive on port", "send from port", "send to address", "send to port": Value Change {
            n230 = event-data() -> ()  [unwired: 1 in, 6 out]
            n231 = call "get paired node.vi"("editor in"=w507) -> ("error out"=w504:errorcluster, "paired node"=w505:refnum<data-value>, "editor out"=w506:refnum<data-value>)  [unwired: 8 in]
            n232 = case shown="No Error" w504 {
              selector: w504 -> [_ w531]
              tunnel: [w513 w531] -> w508
              tunnel: w506 -> [w512 _]
              tunnel: w505 -> [w511 _]
              frame No Error {
                n233 = in-place {
                  in-place-border: [w522] -> w513
                  n234 = in-place-dvr #25(w512) -> (w530:refnum<class "TEC editor node.lvclass">, w525:errorcluster)
                  n235 = in-place-dvr #26(w511) -> (w518:refnum<class "TEC editor node.lvclass">, w516:errorcluster)
                  n236 = Unbundle By Name(w530) -> ("TEC configuration"=w529:refnum<class "TEC configuration.lvclass">)
                  n237 = Unbundle By Name(w518) -> ("TEC configuration"=w520:refnum<class "TEC configuration.lvclass">)
                  n238 = property class="UDP Broadcaster Configuration"(reference=w529, error in=w525, "data access:receive on port"="receive on port", "data access:send from port"="send from port", "data access:send to address"="send to address", "data access:send to port"="send to port") -> (reference out=w528:refnum<class "TEC configuration.lvclass">, error out=w526:errorcluster)
                  n239 = property class="UDP Broadcaster Configuration"(reference=w520, error in=w516, "data access:receive on port"="send to port", "data access:send to port"="receive on port") -> (reference out=w521:refnum<class "TEC configuration.lvclass">, error out=w517:errorcluster)
                  n240 = Bundle By Name(cluster=w530, "TEC configuration"=w528) -> (w527:refnum<class "TEC editor node.lvclass">)
                  n241 = Bundle By Name(cluster=w518, "TEC configuration"=w521) -> (w519:refnum<class "TEC editor node.lvclass">)
                  n242 = Merge Errors(w526, w517) -> (w522:errorcluster)
                  n243 = in-place-dvr #25(w527) -> (w509:errorcluster)  [unwired: 1 out]
                  n244 = in-place-dvr #26(w519) -> (w510:errorcluster)  [unwired: 1 out]
                }
                n245 = flat-sequence {
                  tunnel: w510 -> [_]
                  tunnel: w509 -> [_]
                  frame #0 {
                  }
                }
              }
              frame Error {
              }
            }
          }
          event "Estimated Received Array Size (bytes)": Value Change {
            n246 = event-data() -> ()  [unwired: 1 in, 6 out]
            n247 = in-place {
              in-place-border: [w537] -> w535
              in-place-border: "Estimated Received Array Size (bytes)" -> [w536]
              n248 = in-place-dvr #27(w534) -> (w539:refnum<class "TEC editor node.lvclass">, w538:errorcluster)
              n249 = Unbundle By Name(w539) -> ("TEC configuration"=w541:refnum<class "TEC configuration.lvclass">)
              n250 = property class="UDP Broadcaster Configuration"(reference=w541, error in=w538, "data access:estimated array size"=w536) -> (reference out=w542:refnum<class "TEC configuration.lvclass">, error out=w537:errorcluster)
              n251 = Bundle By Name(cluster=w539, "TEC configuration"=w542) -> (w540:refnum<class "TEC editor node.lvclass">)
              n252 = in-place-dvr #27(w540) -> (w533:errorcluster)  [unwired: 1 out]
            }
            n253 = flat-sequence {
              tunnel: w533 -> [_]
              frame #0 {
              }
            }
          }
        }
        n254 = case shown="Error" w71 {
          selector: w71 -> [w74 w78]
          tunnel: [w75 w79] -> w70
          tunnel: w69 -> [w75 w79]
          tunnel: [w74 w76] -> w68
          frame No Error {
          }
          frame Error {
            n255 = call <vilib>:"Simple Error Handler.vi"("error in (no error)"=w78) -> ("error out"=w77:errorcluster)  [unwired: 4 in, 4 out]
            n256 = call <vilib>:"Clear Errors.vi"("error in (no error)"=w77) -> ("error out"=w76:errorcluster)  [unwired: 6 in]
          }
        }
      }
    }
    frame Error {
    }
  }
  n257 = Unregister For Events(event registration refnum=w47, error in=w46) -> (error out=w43:errorcluster)
  n258 = call <vilib>:"Simple Error Handler.vi"("error in (no error)"=w43) -> ()  [unwired: 4 in, 5 out]
